vi "Initialise Master.vi"(8 "error in (no error)":errorcluster, 11 "MB_TCP in":refnum<class "MB_TCP.lvclass">) -> (0 "error out":errorcluster, 3 "MB_TCP out":refnum<class "MB_TCP.lvclass">)   [LabVIEW 2019, in "MB_TCP.lvclass"]
uses:
  MB_TCP.lvclass
  NI_modbus_upd/TCP/tcp timeouts.ctl
  MB_TCP.lvclass/MB_TCP.ctl
  NI_modbus_upd/TCP/TCP.lvclass/TCP.ctl
  NI_modbus_upd/TCP/TCP.lvclass
  ICPCON Param/ICPCON_Param.lvlib
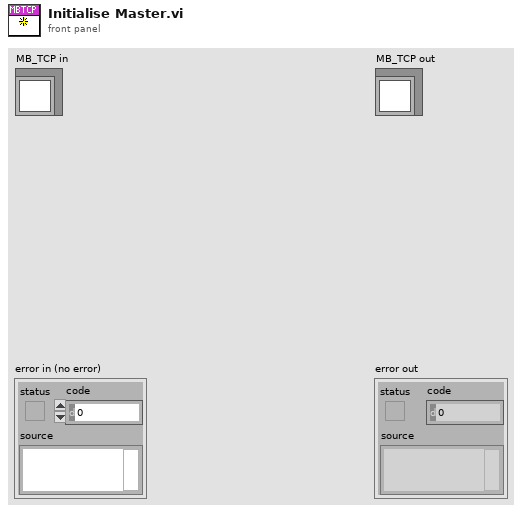
[diagram p1: front panel]
types:
  T1 = typedef "TCP.lvclass/tcp timeouts.ctl" = cluster{"connect timeout":i32, "write timeout":i32, "read timeout":i32}
  T2 = typedef "ICPCON_Param.lvlib/ICPCON Param.ctl" = cluster{"IP addr":refnum<data-value>, "MVIName":refnum<data-value>, "timeouts":refnum<data-value>, "modified":refnum<data-value>}
  T3 = cluster{"Remote IP Address":string, "Remote Port":u16}
  T4 = typedef "ICPCON_Param.lvlib/Eth timeouts.ctl" = cluster{"conn_timeout":i32, "reconn_timeout":i32, "N attempt max":i32, "t_reset_TTL":i32, "write_timeout":i32, "read_timeout":i32, "period":i32}
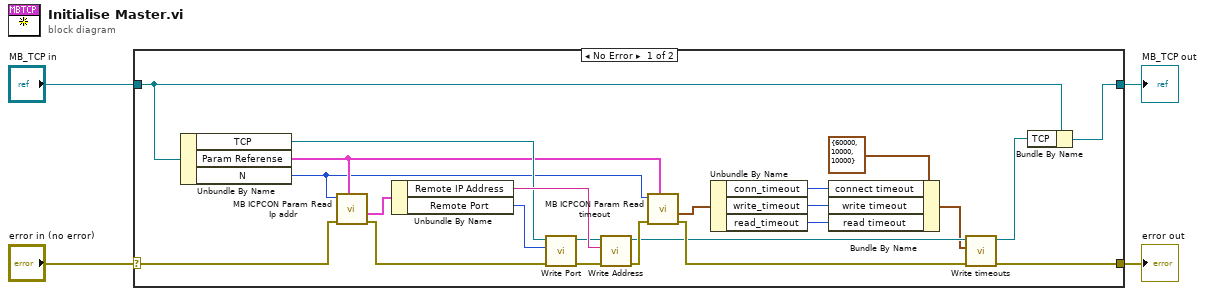
[diagram p0: block diagram]
diagram:
  n1 = case shown="No Error" "error in (no error)" {
    selector: "error in (no error)" -> [w27 w28]
    tunnel: [w5 w28] -> w3
    tunnel: [w19 w29] -> w1
    tunnel: "MB_TCP in" -> [w20 w29]
    frame No Error {
      n2 = Unbundle By Name(w20) -> ("TCP"=w18:refnum<class "TCP.lvclass">, "Param Referense"=w17:T2, "N"=w15:i32)
      n3 = call "MB ICPCON Param Read Ip addr.vi"("Param Reference"=w17, "error in (no error)"=w27, "N"=w15) -> ("error out"=w21:errorcluster, "IP address"=w26:T3)  [unwired: 7 in]
      n4 = Unbundle By Name(w26) -> ("Remote IP Address"=w25:string, "Remote Port"=w24:u16)
      n5 = call "Write Port.vi"("error in (no error)"=w21, "port"=w24, "TCP in"=w18) -> ("error out"=w22:errorcluster, "TCP out"=w23:refnum<class "TCP.lvclass">)  [unwired: 7 in]
      n6 = call "Write Address.vi"("error in (no error)"=w22, "address"=w25, "TCP in"=w23) -> ("error out"=w16:errorcluster, "TCP out"=w8:refnum<class "TCP.lvclass">)  [unwired: 7 in]
      n7 = call "MB ICPCON Param Read timeout.vi"("Param Reference"=w17, "error in (no error)"=w16, "N"=w15) -> ("error out"=w14:errorcluster, "timeout"=w13:T4)  [unwired: 7 in]
      n8 = Unbundle By Name(w13) -> ("conn_timeout"=w12:i32, "write_timeout"=w10:i32, "read_timeout"=w9:i32)
      n9 = Bundle By Name(cluster=T1 {"connect timeout"=60000, "write timeout"=10000, "read timeout"=10000} ("timeouts"), "connect timeout"=w12, "write timeout"=w10, "read timeout"=w9) -> (w7:T1)
      n10 = call "Write timeouts.vi"("error in (no error)"=w14, "timeouts"=w7, "TCP Master in"=w8) -> ("error out"=w5:errorcluster, "TCP Master out"=w6:refnum<class "TCP.lvclass">)  [unwired: 7 in]
      n11 = Bundle By Name(cluster=w20, "TCP"=w6) -> (w19:refnum<class "MB_TCP.lvclass">)
    }
    frame Error {
    }
  }
  "error out" <- w3
  "MB_TCP out" <- w1
